vi "File Changed Callback.vi"(4 "用户参数":variant, 5 "事件数据":cluster{"sender":refnum<k24>, "e":refnum<k24>}, 6 "控件引用":refnum<k24>, 7 "事件通用数据":cluster{"事件源":i32, "事件类型":u32, "时间标识":u32}) -> ()   [LabVIEW 2012, in "FileSystem Watcher.lvlib"]
uses:
  FileSystem Watcher.lvlib
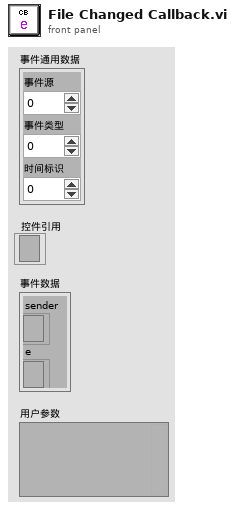
[diagram p1: front panel]
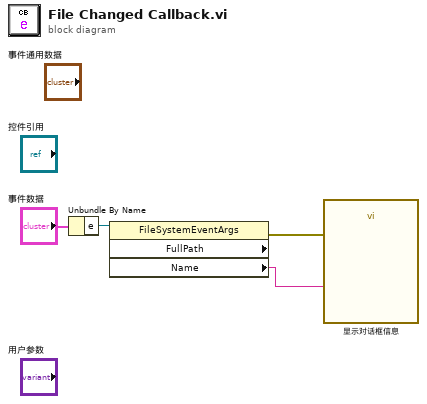
[diagram p0: block diagram]
diagram:
  n1 = Unbundle By Name("事件数据") -> ("e"=w3:refnum<k24>)
  n2 = property class="FileSystemEventArgs" props=["FullPath", "Name"](reference=w3) -> (error out=w2:errorcluster, "Name"=w1:string)  [unwired: 1 in, 2 out]
  n3 = call "显示对话框信息"("error in (no error)"=w2, "Message"=w1) -> ()  [unwired: 8 in, 2 out]
